vi "Path配置.vi"() -> (2 "确定":bool)   [LabVIEW 2020]
uses:
  Global.vi
  <vilib>/Utility/file.llb/Write Delimited Spreadsheet (string).vi
panel:
  in  "Path":string="D:\\MES"
  in  "取消":bool
  in  "确定":bool
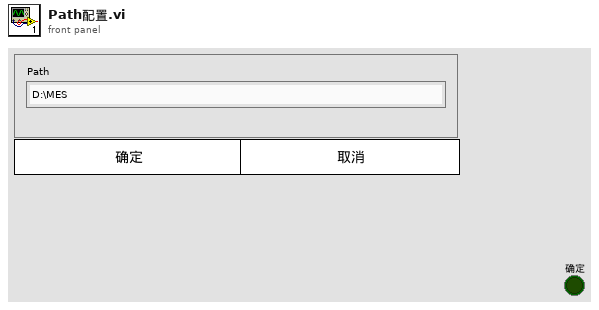
[diagram p1: front panel]
types:
  T1 = cluster{"Server":string, "audit_mode":string, "tsid":string, "model":string, "product":string, "test_station":string, "station_id":string, "test_station_name":string, "Webservice":string}
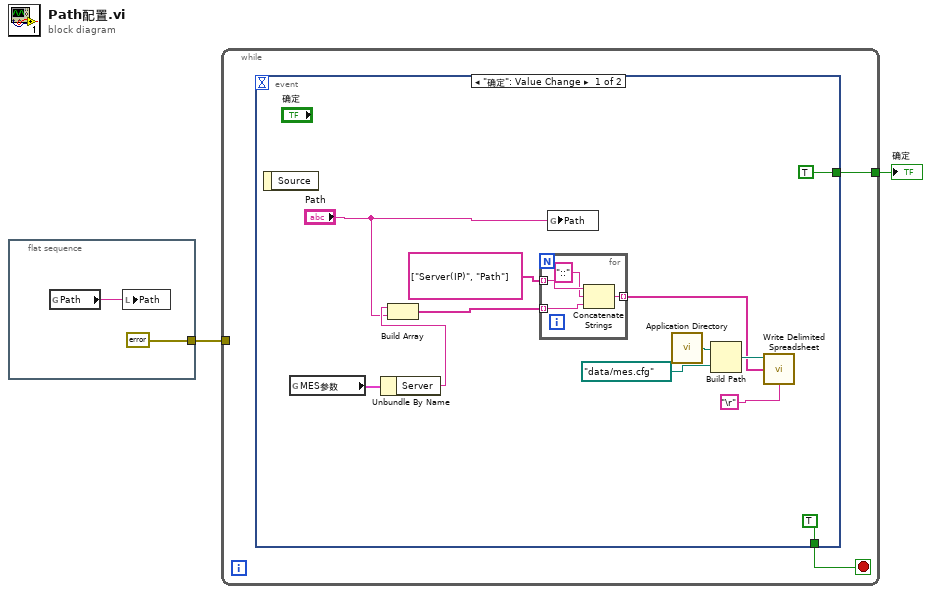
[diagram p0: block diagram]
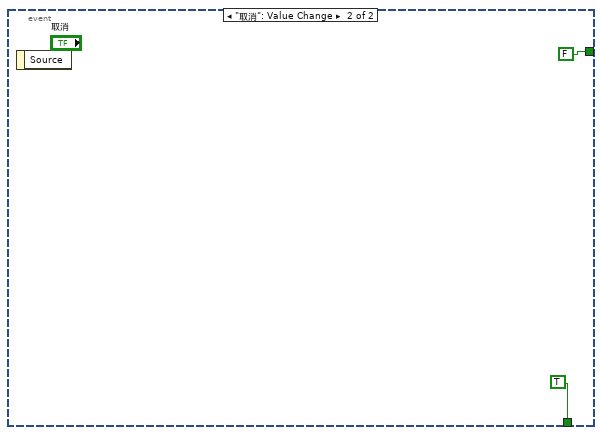
[diagram p2: hidden frame]
diagram:
  n1 = flat-sequence {
    tunnel: [errorcluster {"status"=FALSE, "code"=0, "source"=""} ("错误常量")] -> w1
    frame #0 {
      n2 = global read "Global.vi" "Path"() -> (w3:string)
      n3 = local write "Path"(w3) -> ()
    }
  }
  n4 = while {
    tunnel: [w5] -> w2
    tunnel: w1 -> [_]
    stop <- w6 stop-if-true
    n5 = event shown="[0] \"确定\": Value Change" {
      selector: _ -> [_ _]
      dyn-events: _ -> [_ _]
      timeout: _ -> [_ _]
      tunnel: [TRUE TRUE] -> w6
      tunnel: [TRUE FALSE] -> w5
      event "确定": Value Change {
        n6 = event-data() -> ()  [unwired: 1 in, 1 out]
        n7 = global read "Global.vi" "MES参数"() -> (w9:T1)
        n8 = Unbundle By Name(w9) -> ("Server"=w8:string)
        n9 = Build Array(w8, "Path") -> (w12:string[])
        n10 = for {
          tunnel: string[] ["Server(IP)", "Path"] ("转置的数组") -> [w22] mode=indexing
          tunnel: w12 -> [w20] mode=indexing
          tunnel: [w19] -> w11 mode=indexing
          n11 = Concatenate Strings(w22, "::" ("String"), w20) -> (w19:string)
        }
        n12 = global write "Global.vi" "Path"("Path") -> ()
        n13 = call <vilib>:"Application Directory.vi"() -> ("Application Directory"=w15:path)
        n14 = Build Path(base path=w15, name or relative path=path "data/mes.cfg") -> (appended path=w14:path)
        n15 = call-poly <vilib>:"Write Delimited Spreadsheet.vi"("file path (dialog if empty)"=w14, "1D data"=w11, "delimiter (\\t)"="\r") -> ()  [unwired: 11 in, 2 out]
      }
      event "取消": Value Change {
        n16 = event-data() -> ()  [unwired: 1 in, 1 out]
      }
    }
  }
  "确定" <- w2
